vi "Launch Monitor Process.vi"(8 "error in (no error)":errorcluster, 10 "TopLevel":refnum<class "TopLevel.lvclass">, 11 "DAQ":refnum<class "DAQ.lvclass">) -> (0 "error out":errorcluster, 3 "DAQ":refnum<class "DAQ.lvclass">)   [LabVIEW 2022 SP3, in "DAQ.lvclass"]
doc: "Developed by Kevin Thompson\nkevin@thompsonengineering.net\n\nCopyright 2018-2020\nThompson Engineering, LLC"
uses:
  DAQ.lvclass
  TopLevel/TopLevel.lvclass
  MonitoringProcess_DAQ.vi
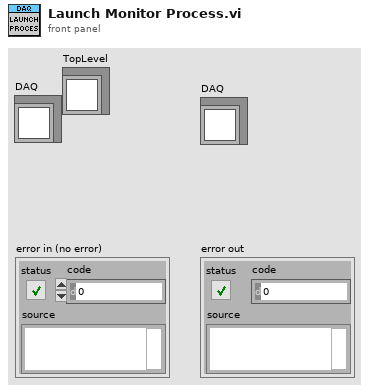
[diagram p1: front panel]
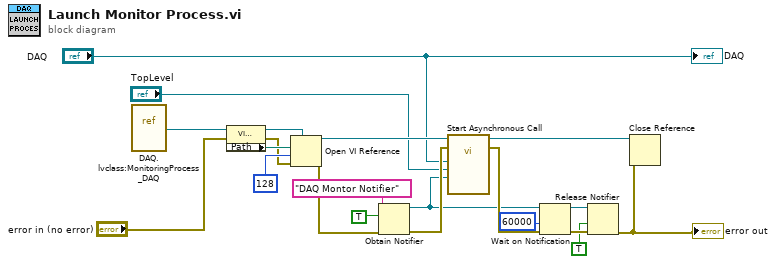
[diagram p0: block diagram]
diagram:
  n1 = vi-ref "DAQ.lvclass:MonitoringProcess_DAQ.vi"() -> (w19:refnum<vi>)
  n2 = property class="VI (strict)"(reference=w19, error in="error in (no error)") -> (reference out=w17:refnum<vi>, error out=w10:errorcluster, "Path"=w18:path)
  n3 = Open VI Reference(type specifier VI Refnum (for type only)=w17, vi path=w18, options=128, error in (no error)=w10) -> (vi reference=w15:refnum<vi>, error out=w11:errorcluster)  [unwired: 2 in]
  n4 = Obtain Notifier(name (unnamed)="DAQ Montor Notifier", notification data type=TRUE, error in (no error)=w11) -> (notifier out=w8:refnum<notifier>, error out=w13:errorcluster)  [unwired: 1 in, 1 out]
  n5 = call-by-ref "Start Asynchronous Call"(reference=w15, error in=w13, "start process sync notifier"=w8, "TopLevel"="TopLevel", "DAQ"="DAQ") -> (reference out=w5:refnum<vi>, error out=w12:errorcluster)  [unwired: 8 in, 1 out]
  n6 = Wait on Notification(notifier=w8, timeout in ms (-1)=60000, error in (no error)=w12) -> (notifier out=w6:refnum<notifier>, error out=w7:errorcluster)  [unwired: 1 in, 2 out]
  n7 = Release Notifier(notifier=w6, force destroy? (F)=TRUE, error in (no error)=w7) -> (error out=w21:errorcluster)  [unwired: 2 out]
  "error out" <- w21
  n8 = Close Reference(reference=w5, error in (no error)=w21) -> ()  [unwired: 1 out]
  "DAQ" <- "DAQ"
